vi "RydbergExpControl_2014.09.17_beta_b.vi"() -> ()   [LabVIEW 2013]
uses:
  AndorCamera/camera_controls.ctl
  <userlib>/atmcd32d.llb/AcquisitionMode_mode typedef.ctl
  <userlib>/atmcd32d.llb/TriggerMode_mode typedef.ctl
  6704/6704_static_voltages_control.ctl
  rydberg_state_machine_states.ctl
panel:
  out "Current Param Value":dbl
  out "Camera Ready":bool
  out "Exp Running":bool
  out "error out":errorcluster
  in  "Trigger Snap Mode":bool
  in  "Shutdown Experiment":bool
  in  "Start Experiment":bool
  out "Started in trigger snap":bool=TRUE
  out "Waveform Chart":dbl(graph)
  in  "Count Number?":bool
  out "Number":dbl format="%^#_6g"
  out "OD":dbl[][](graph)
  out "Atom Closeup":dbl[][](graph)
  out "Atoms - BG":dbl[][](graph)
  out "Background Image":dbl[][](graph)
  out "Atom Image":dbl[][](graph)
  in  "Tab Control":T1(tab)
  in  "Instructions":T2(array[cluster])=[{"Instruct Data"=0, "Op Code"=0, "Flags"=[TRUE, FALSE, FALSE, FALSE, FALSE, FALSE, FALSE, FALSE, FALSE, FALSE, FALSE, FALSE, FALSE, FALSE, FALSE, FALSE, FALSE, FALSE, FALSE, FALSE, FALSE, FALSE, FALSE, FALSE], "Comments"="", "Time (s)"=0.1}, {"Instruct Data"=0, "Op Code"=0, "Flags"=[FALSE, FALSE, FALSE, FALSE, FALSE, FALSE, FALSE, FALSE, FALSE, FALSE, FALSE, FALSE, FALSE, FALSE, FALSE, FALSE, FALSE, FALSE, FALSE, FALSE, FALSE, FALSE, FALSE, FALSE], "Comments"="", "Time (s)"=0.1}, {"Instruct Data"=0, "Op Code"=0, "Flags"=[TRUE, FALSE, FALSE, FALSE, FALSE, FALSE, FALSE, FALSE, FALSE, FALSE, FALSE, FALSE, FALSE, FALSE, FALSE, FALSE, FALSE, FALSE, FALSE, FALSE, FALSE, FALSE, FALSE, FALSE], "Comments"="", "Time (s)"=0.1}, {"Instruct Data"=0, "Op Code"=6, "Flags"=[FALSE, FALSE, FALSE, FALSE, FALSE, FALSE, FALSE, FALSE, FALSE, FALSE, FALSE, FALSE, FALSE, FALSE, FALSE, FALSE, FALSE, FALSE, FALSE, FALSE, FALSE, FALSE, FALSE, FALSE], "Comments"="", "Time (s)"=0.1}] {"Time (s)" format="%.3p"; "Op Code" items=["Continue", "Stop", "Loop", "End Loop", "JSR", "RTS", "Branch", "Long Delay", "Wait"]}
  in  "Parameter Nickname (no spaces)":string[](array[string])
  in  "Number of Parameters to Scan":i32=1 min=1
  in  "Channels to Change":dbl[](array[numeric])=[0.0, 0.0, 0.0]
  in  "Parameters to Change":enum16{"PulseBlaster", "Static Voltage"}[](array[ring])=[enum."Static Voltage", enum."Static Voltage", enum."Static Voltage"]
  in  "Step Sizes":dbl[](array[numeric])=[0.0, 0.0, 0.0]
  in  "Final Values":dbl[](array[numeric])=[0.0, 0.0, 0.0]
  in  "Initial Values":dbl[](array[numeric])
  in  "Scan Base Name":string
  in  "Raw_Data Folder":path
  out "Full Scan Name":string
  out "Camera Information":T3 {"VS Speed (us)" format="%.2f"}
  in  "Acquisition Parameters":T4={"Acquisition Mode"=enum."Kinetics", "Trigger Mode"=enum."External", "Frame \nTransfer"=FALSE, "Exposure Time (s)"=0.0001, "Accumulation Cycle Time (s)"=0.0, "# Accumulations"=1, "# Kinetics"=2, "Kinetic Cycle Time (s)"=0.0, "Horizontal Bin Size"=1, "Vertical Bin Size"=1} {"Vertical Bin Size" min=1; "Horizontal Bin Size" min=1; "Kinetic Cycle Time (s)" format="%.2f"; "# Kinetics" min=1; "# Accumulations" min=1; "Accumulation Cycle Time (s)" format="%.2f"; "Exposure Time (s)" format="%.2e"}
  out "Calcualted Times":T7 {"Kinetic" format="%.4f"; "Accumulate" format="%.4f"; "Exposure" format="%.4f"}
  in  "Red MOT 87 Inputs":T8={"Active Device"="6733_Red_87", "Active Channels"=[TRUE, FALSE, FALSE, FALSE, FALSE, FALSE, FALSE, FALSE], "Waveform Parameters"=[[{"Functional Form"=enum."Polynomial", "Start Voltage"=0.0, "End Voltage"=0.0, "Time"=0.0, "Degree"=1, "Sample Rate"=0.0}, {"Functional Form"=enum."Exponential", "Start Voltage"=0.0, "End Voltage"=0.0, "Time"=0.0, "Degree"=1, "Sample Rate"=0.0}, {"Functional Form"=enum."Exponential", "Start Voltage"=0.0, "End Voltage"=0.0, "Time"=0.0, "Degree"=1, "Sample Rate"=0.0}, {"Functional Form"=enum."Exponential", "Start Voltage"=0.0, "End Voltage"=0.0, "Time"=0.0, "Degree"=1, "Sample Rate"=0.0}, {"Functional Form"=enum."Exponential", "Start Voltage"=0.0, "End Voltage"=0.0, "Time"=0.0, "Degree"=1, "Sample Rate"=0.0}, {"Functional Form"=enum."Exponential", "Start Voltage"=0.0, "End Voltage"=0.0, "Time"=0.0, "Degree"=1, "Sample Rate"=0.0}], [{"Functional Form"=enum."Exponential", "Start Voltage"=0.0, "End Voltage"=0.0, "Time"=0.0, "Degree"=1, "Sample Rate"=0.0}, {"Functional Form"=enum."Exponential", "Start Voltage"=0.0, "End Voltage"=0.0, "Time"=0.0, "Degree"=1, "Sample Rate"=0.0}, {"Functional Form"=enum."Exponential", "Start Voltage"=0.0, "End Voltage"=0.0, "Time"=0.0, "Degree"=1, "Sample Rate"=0.0}, {"Functional Form"=enum."Exponential", "Start Voltage"=0.0, "End Voltage"=0.0, "Time"=0.0, "Degree"=1, "Sample Rate"=0.0}, {"Functional Form"=enum."Exponential", "Start Voltage"=0.0, "End Voltage"=0.0, "Time"=0.0, "Degree"=1, "Sample Rate"=0.0}, {"Functional Form"=enum."Exponential", "Start Voltage"=0.0, "End Voltage"=0.0, "Time"=0.0, "Degree"=1, "Sample Rate"=0.0}], [{"Functional Form"=enum."Exponential", "Start Voltage"=0.0, "End Voltage"=0.0, "Time"=0.0, "Degree"=1, "Sample Rate"=0.0}, {"Functional Form"=enum."Exponential", "Start Voltage"=0.0, "End Voltage"=0.0, "Time"=0.0, "Degree"=1, "Sample Rate"=0.0}, {"Functional Form"=enum."Exponential", "Start Voltage"=0.0, "End Voltage"=0.0, "Time"=0.0, "Degree"=1, "Sample Rate"=0.0}, {"Functional Form"=enum."Exponential", "Start Voltage"=0.0, "End Voltage"=0.0, "Time"=0.0, "Degree"=1, "Sample Rate"=0.0}, {"Functional Form"=enum."Exponential", "Start Voltage"=0.0, "End Voltage"=0.0, "Time"=0.0, "Degree"=1, "Sample Rate"=0.0}, {"Functional Form"=enum."Exponential", "Start Voltage"=0.0, "End Voltage"=0.0, "Time"=0.0, "Degree"=1, "Sample Rate"=0.0}], [{"Functional Form"=enum."Exponential", "Start Voltage"=0.0, "End Voltage"=0.0, "Time"=0.0, "Degree"=1, "Sample Rate"=0.0}, {"Functional Form"=enum."Exponential", "Start Voltage"=0.0, "End Voltage"=0.0, "Time"=0.0, "Degree"=1, "Sample Rate"=0.0}, {"Functional Form"=enum."Exponential", "Start Voltage"=0.0, "End Voltage"=0.0, "Time"=0.0, "Degree"=1, "Sample Rate"=0.0}, {"Functional Form"=enum."Exponential", "Start Voltage"=0.0, "End Voltage"=0.0, "Time"=0.0, "Degree"=1, "Sample Rate"=0.0}, {"Functional Form"=enum."Exponential", "Start Voltage"=0.0, "End Voltage"=0.0, "Time"=0.0, "Degree"=1, "Sample Rate"=0.0}, {"Functional Form"=enum."Exponential", "Start Voltage"=0.0, "End Voltage"=0.0, "Time"=0.0, "Degree"=1, "Sample Rate"=0.0}], [{"Functional Form"=enum."Exponential", "Start Voltage"=0.0, "End Voltage"=0.0, "Time"=0.0, "Degree"=1, "Sample Rate"=0.0}, {"Functional Form"=enum."Exponential", "Start Voltage"=0.0, "End Voltage"=0.0, "Time"=0.0, "Degree"=1, "Sample Rate"=0.0}, {"Functional Form"=enum."Exponential", "Start Voltage"=0.0, "End Voltage"=0.0, "Time"=0.0, "Degree"=1, "Sample Rate"=0.0}, {"Functional Form"=enum."Exponential", "Start Voltage"=0.0, "End Voltage"=0.0, "Time"=0.0, "Degree"=1, "Sample Rate"=0.0}, {"Functional Form"=enum."Exponential", "Start Voltage"=0.0, "End Voltage"=0.0, "Time"=0.0, "Degree"=1, "Sample Rate"=0.0}, {"Functional Form"=enum."Exponential", "Start Voltage"=0.0, "End Voltage"=0.0, "Time"=0.0, "Degree"=1, "Sample Rate"=0.0}], [{"Functional Form"=enum."Exponential", "Start Voltage"=0.0, "End Voltage"=0.0, "Time"=0.0, "Degree"=1, "Sample Rate"=0.0}, {"Functional Form"=enum."Exponential", "Start Voltage"=0.0, "End Voltage"=0.0, "Time"=0.0, "Degree"=1, "Sample Rate"=0.0}, {"Functional Form"=enum."Exponential", "Start Voltage"=0.0, "End Voltage"=0.0, "Time"=0.0, "Degree"=1, "Sample Rate"=0.0}, {"Functional Form"=enum."Exponential", "Start Voltage"=0.0, "End Voltage"=0.0, "Time"=0.0, "Degree"=1, "Sample Rate"=0.0}, {"Functional Form"=enum."Exponential", "Start Voltage"=0.0, "End Voltage"=0.0, "Time"=0.0, "Degree"=1, "Sample Rate"=0.0}, {"Functional Form"=enum."Exponential", "Start Voltage"=0.0, "End Voltage"=0.0, "Time"=0.0, "Degree"=1, "Sample Rate"=0.0}], [{"Functional Form"=enum."Exponential", "Start Voltage"=0.0, "End Voltage"=0.0, "Time"=0.0, "Degree"=1, "Sample Rate"=0.0}, {"Functional Form"=enum."Exponential", "Start Voltage"=0.0, "End Voltage"=0.0, "Time"=0.0, "Degree"=1, "Sample Rate"=0.0}, {"Functional Form"=enum."Exponential", "Start Voltage"=0.0, "End Voltage"=0.0, "Time"=0.0, "Degree"=1, "Sample Rate"=0.0}, {"Functional Form"=enum."Exponential", "Start Voltage"=0.0, "End Voltage"=0.0, "Time"=0.0, "Degree"=1, "Sample Rate"=0.0}, {"Functional Form"=enum."Exponential", "Start Voltage"=0.0, "End Voltage"=0.0, "Time"=0.0, "Degree"=1, "Sample Rate"=0.0}, {"Functional Form"=enum."Exponential", "Start Voltage"=0.0, "End Voltage"=0.0, "Time"=0.0, "Degree"=1, "Sample Rate"=0.0}], [{"Functional Form"=enum."Exponential", "Start Voltage"=0.0, "End Voltage"=0.0, "Time"=0.0, "Degree"=1, "Sample Rate"=0.0}, {"Functional Form"=enum."Exponential", "Start Voltage"=0.0, "End Voltage"=0.0, "Time"=0.0, "Degree"=1, "Sample Rate"=0.0}, {"Functional Form"=enum."Exponential", "Start Voltage"=0.0, "End Voltage"=0.0, "Time"=0.0, "Degree"=1, "Sample Rate"=0.0}, {"Functional Form"=enum."Exponential", "Start Voltage"=0.0, "End Voltage"=0.0, "Time"=0.0, "Degree"=1, "Sample Rate"=0.0}, {"Functional Form"=enum."Exponential", "Start Voltage"=0.0, "End Voltage"=0.0, "Time"=0.0, "Degree"=1, "Sample Rate"=0.0}, {"Functional Form"=enum."Exponential", "Start Voltage"=0.0, "End Voltage"=0.0, "Time"=0.0, "Degree"=1, "Sample Rate"=1.0}]], "Active Phases"=[TRUE, FALSE, FALSE, FALSE, FALSE, FALSE], "Phase Times"=[0.001], "Trigger Channel"="/6733_Red_87/PFI0"} {"Phase Times" format="%.0p"; "Waveform Parameters"."Degree" min=1}
  in  "6704 Static Voltage Settings":T9={"Device Name"="6704_Static", "Voltages"=[5.0, 0.0, 0.0, 0.0, 0.0, 0.0, 0.0, 0.0, 0.0, 0.0, 0.0, 0.0, 0.0, 0.0, 0.0, 0.0]}
  out "Andor Initialization Error Codes":T10
  out "Acq. Error Codes":T11
  out "Tree":string(tree)
  # "(1) 461 MOT beams"
  # "(2) Imaging AOM 1"
  # "(3) Imaging AOM 2"
  # "(4) Camera"
  # "(5) Zeeman shutter"
  # "(6) Repumper shutter"
  # "(7) 461 MOT coils"
  # "(8) 689 MOT coils"
  # "(9) 87 Sr Red MOT Trig"
  # "(10) Blue MOT Shutter"
  # "(11) Red AOM"
  # "(12) Sat Abs Current Switch"
  # "(13) Zeeman MOSFET"
  # "1"
  # "2"
  # "3"
  # "4"
  # "5"
  # "6"
  # "7"
  # "8"
  # "9"
  # "10"
  # "11"
  # "12"
  # "13"
  # "14"
  # "15"
  # "16"
  # "17"
  # "18"
  # "19"
  # "20"
  # "21"
  # "22"
  # "23"
  # "24"
  # "Conversion formulae to be added"
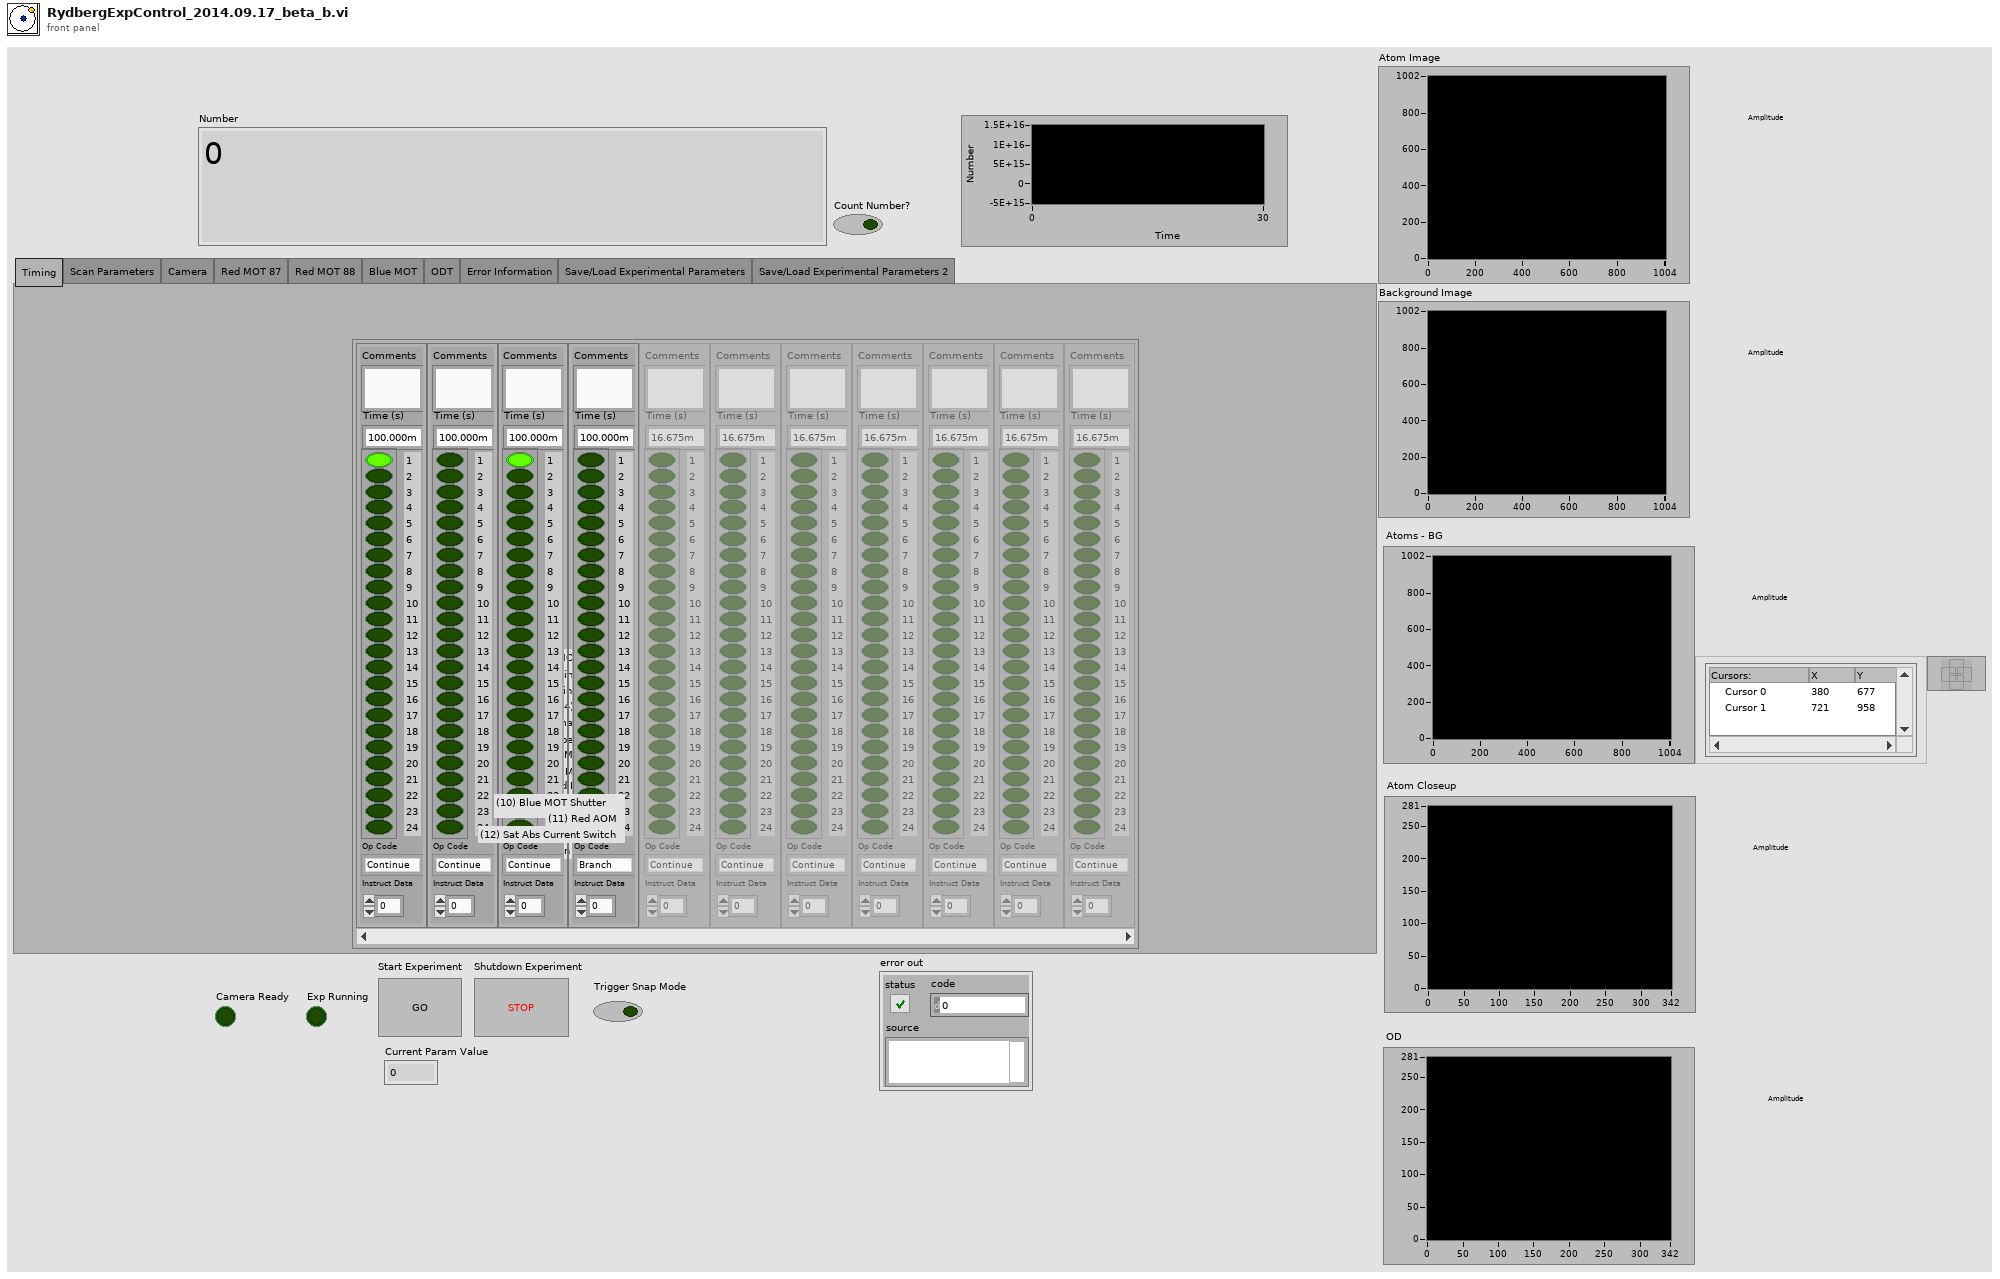
[diagram p1: front panel]
types:
  T1 = enum32{"Timing", "Scan Parameters", "Camera", "Red MOT 87", "Red MOT 88", "Blue MOT", "ODT", "Error Information", "Save/Load Experimental Parameters", "Save/Load Experimental Parameters 2"}
  T2 = cluster{"Instruct Data":i32, "Op Code":i32, "Flags":bool[], "Comments":string, "Time (s)":dbl}[]
  T3 = cluster{"xpixels":i32, "ypixels":i32, "# VS Speeds":i32, "VS Speed (us)":sgl, "Temperature Stable":bool, "Temperature (C)":i32}
  T4 = typedef "camera_controls.ctl" = cluster{"Acquisition Mode":T5, "Trigger Mode":T6, "Frame \nTransfer":bool, "Exposure Time (s)":sgl, "Accumulation Cycle Time (s)":sgl, "# Accumulations":i32, "# Kinetics":i32, "Kinetic Cycle Time (s)":sgl, "Horizontal Bin Size":i32, "Vertical Bin Size":i32}
  T5 = typedef "AcquisitionMode_mode typedef.ctl" = enum16{"Reserved (0)", "Single Scan", "Accumulate", "Kinetics", "Fast Kinetics", "Run Till Abort", "Reserved (6)", "Reserved (7)", "Reserved (8)", "Time Delayed Integration"}
  T6 = typedef "TriggerMode_mode typedef.ctl" = enum16{"Internal", "External", "N/A (2)", "N/A (3)", "N/A (4)", "N/A (5)", "External Start", "External Exposure (Bulb)", "N/A (8)", "External FVB EM", "Software", "N/A (11)", "External Charge Shifting"}
  T7 = cluster{"Exposure":sgl, "Accumulate":sgl, "Kinetic":sgl}
  T8 = cluster{"Active Device":string, "Active Channels":bool[], "Waveform Parameters":cluster{"Functional Form":enum16{"Polynomial", "Exponential"}, "Start Voltage":dbl, "End Voltage":dbl, "Time":dbl, "Degree":i8, "Sample Rate":dbl}[][], "Active Phases":bool[], "Phase Times":dbl[], "Trigger Channel":tag}
  T9 = typedef "6704_static_voltages_control.ctl" = cluster{"Device Name":string, "Voltages":dbl[]}
  T10 = cluster{"Initalize Error Code":u32, "GetDetector Error Code":u32, "Get#VSSpeeds Error Code":u32, "Set VS Speed Error":u32, "CoolerOn Error Code":u32, "GetTemperature Error Code":u32, "Shutdown Error Code":u32}
  T11 = cluster{"Set Acq. Mode Error":u32, "Set Trigger Mode Error":u32, "Set FT Error Code":u32, "Set Exposure Time Error Code":u32, "Set Accum Time Error":u32, "Set # Accum Error":u32, "Set # Kinetics Error":u32, "SetKinCycleTime Error":u32}
  T12 = typedef "rydberg_state_machine_states.ctl" = enum16{"Initialize", "Idle", "Experiment Running", "Trigger Snap Mode", "Scan Mode", "Load Experiment", "Shutdown"}
  T13 = cluster{"6704 Static Voltage Settings":T9, "Instructions":cluster{"Instruct Data":i32, "Op Code":i32, "Flags":bool[], "Comments":string, "Time (s)":dbl}[], "Red MOT 87 Inputs":cluster{"Active Device":string, "Active Channels":bool[], "Waveform Parameters":cluster{"Functional Form":enum16{"Polynomial", "Exponential"}, "Start Voltage":dbl, "End Voltage":dbl, "Time":dbl, "Degree":i8, "Sample Rate":dbl}[][], "Active Phases":bool[], "Phase Times":dbl[], "Trigger Channel":tag}}
  T14 = cluster{"Initial Values":refnum<vi>, "Channels to Change":refnum<vi>, "Final Values":refnum<vi>, "Step Sizes":refnum<vi>}
  T15 = typedef "LVCursorListTypeDef.ctl" = cluster{"Name":string, "Color":u32, "Style":u8, "Point Style":u8, "Name Visible":bool, "Allow Drag":bool, "Cursor Mode":u32, "Plot":i32, "Index":i32, "Position":cluster{"X":dbl, "Y":dbl}, "X Scale":u32, "Y Scale":u32, "Watch Plots":i32[], "Watch All Plots":bool, "Plot Area":i32, "Label Offset":cluster{"X":dbl, "Y":dbl}}[]
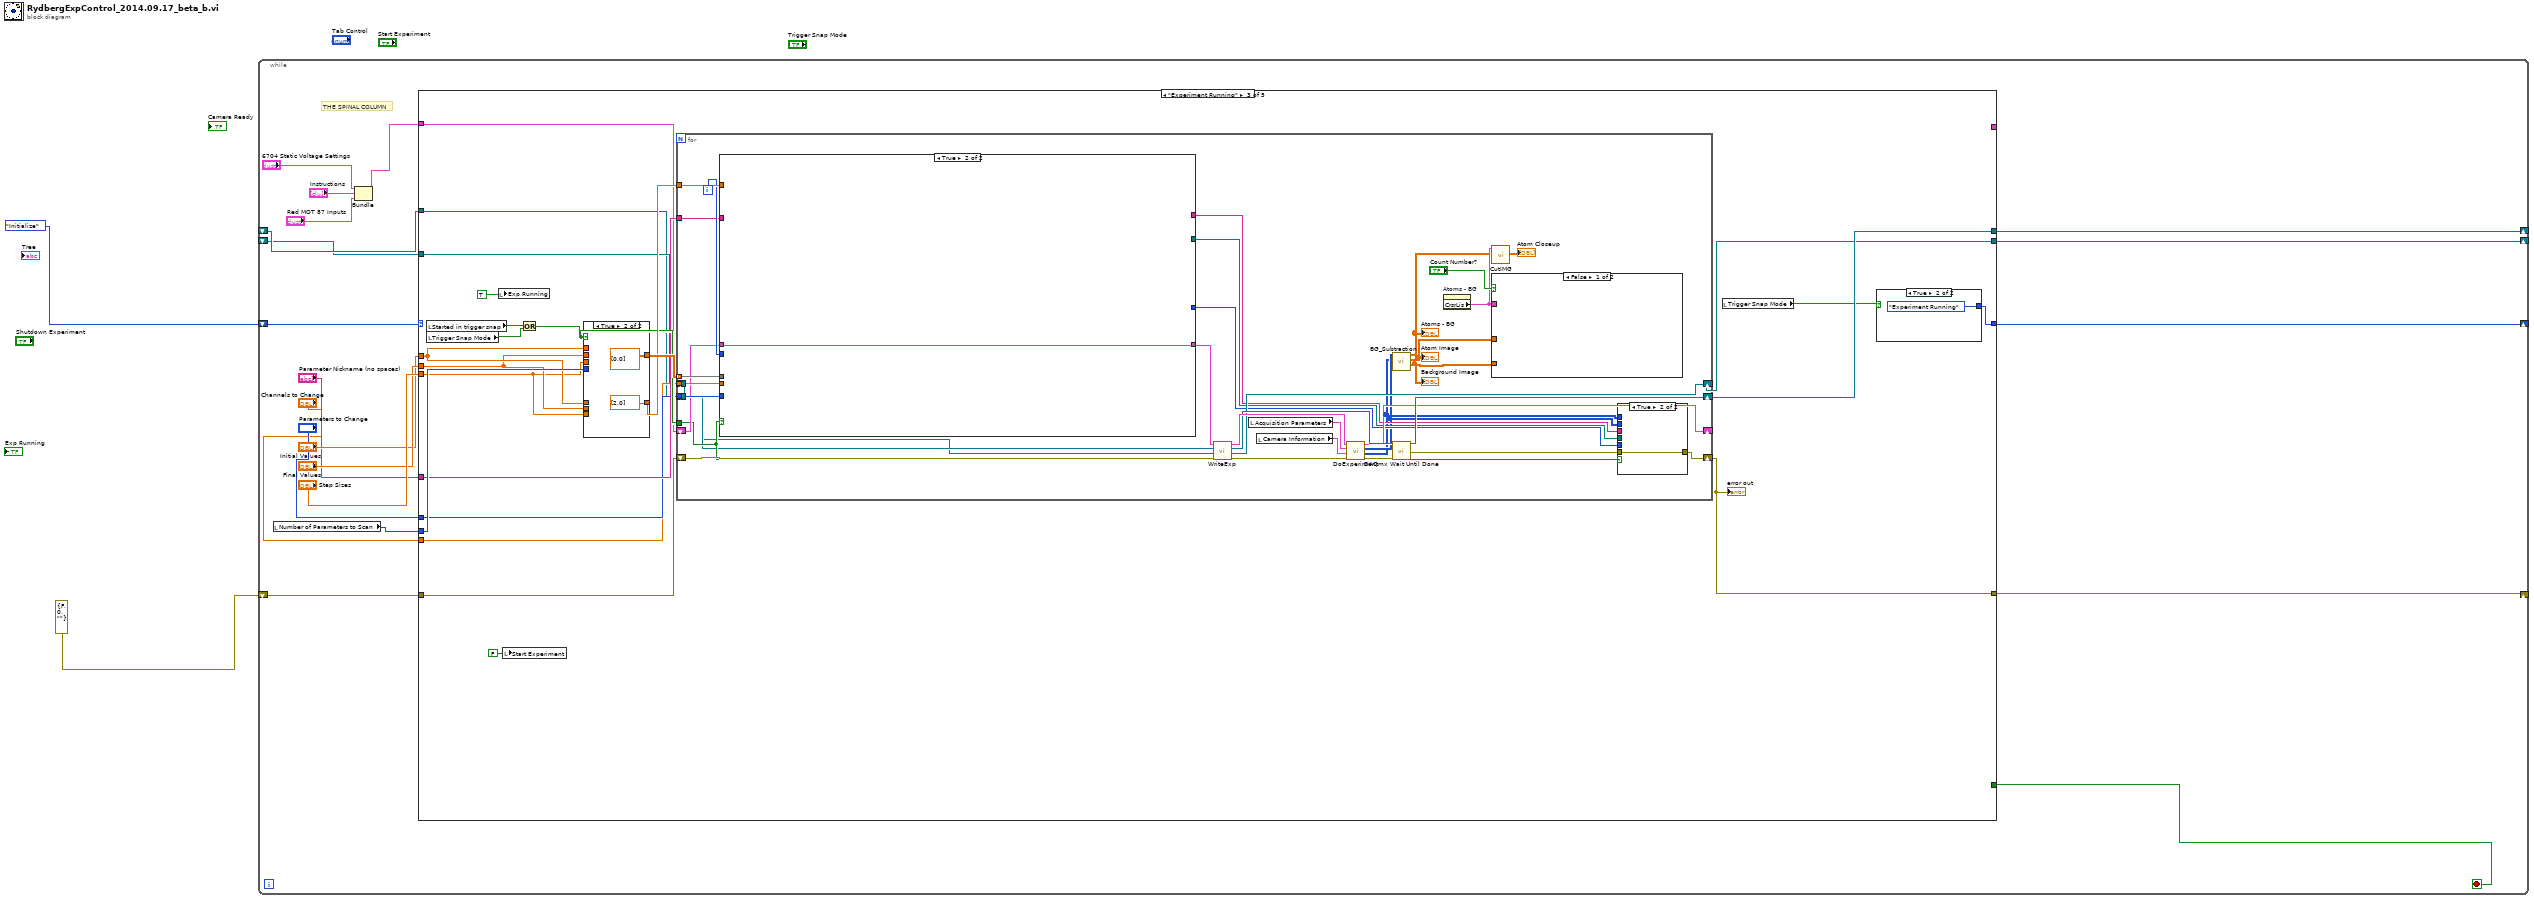
[diagram p0: block diagram]
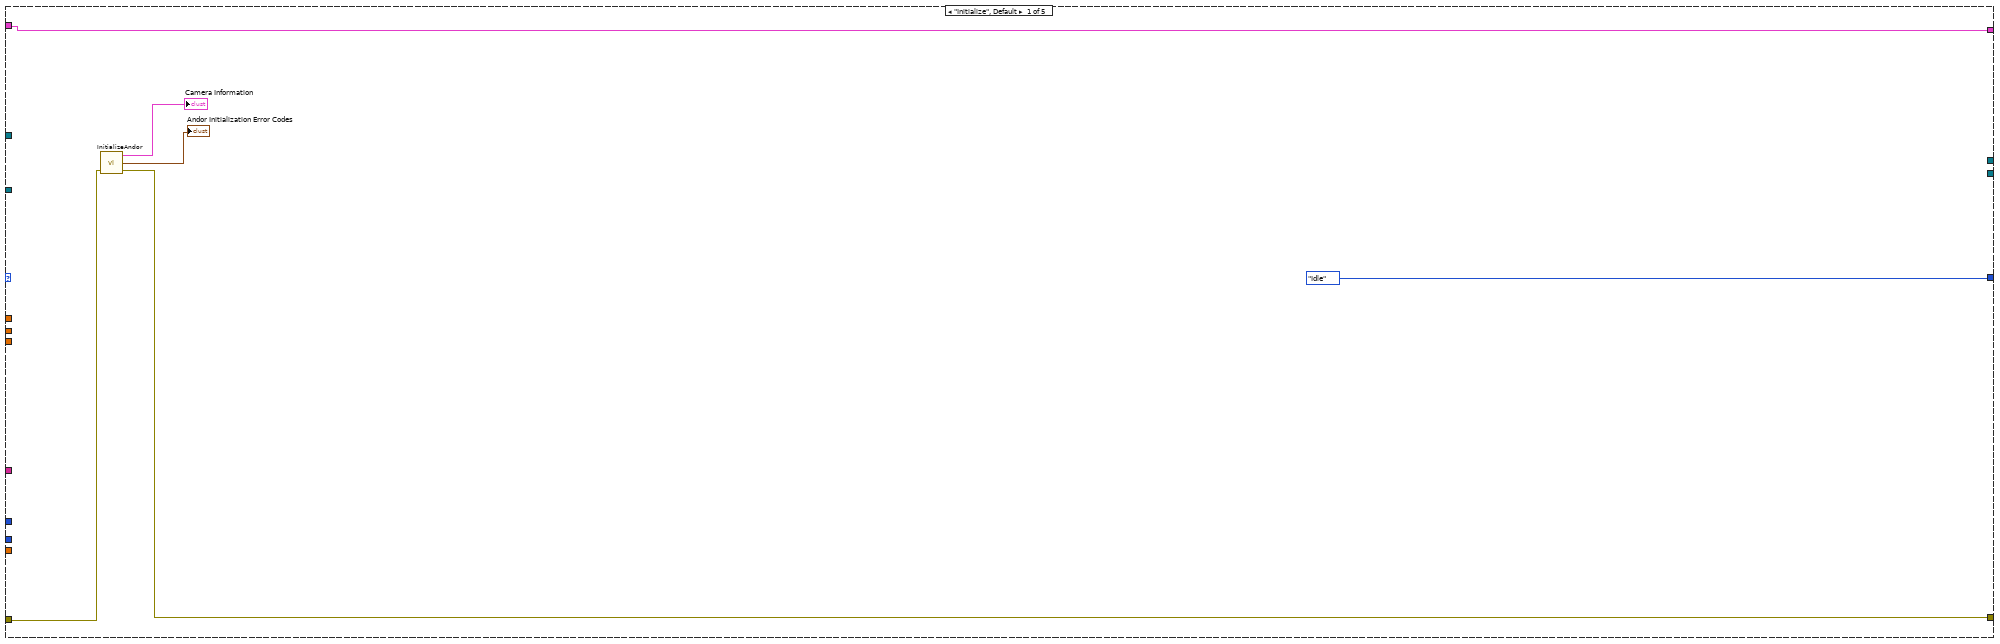
[diagram p2: hidden frame]
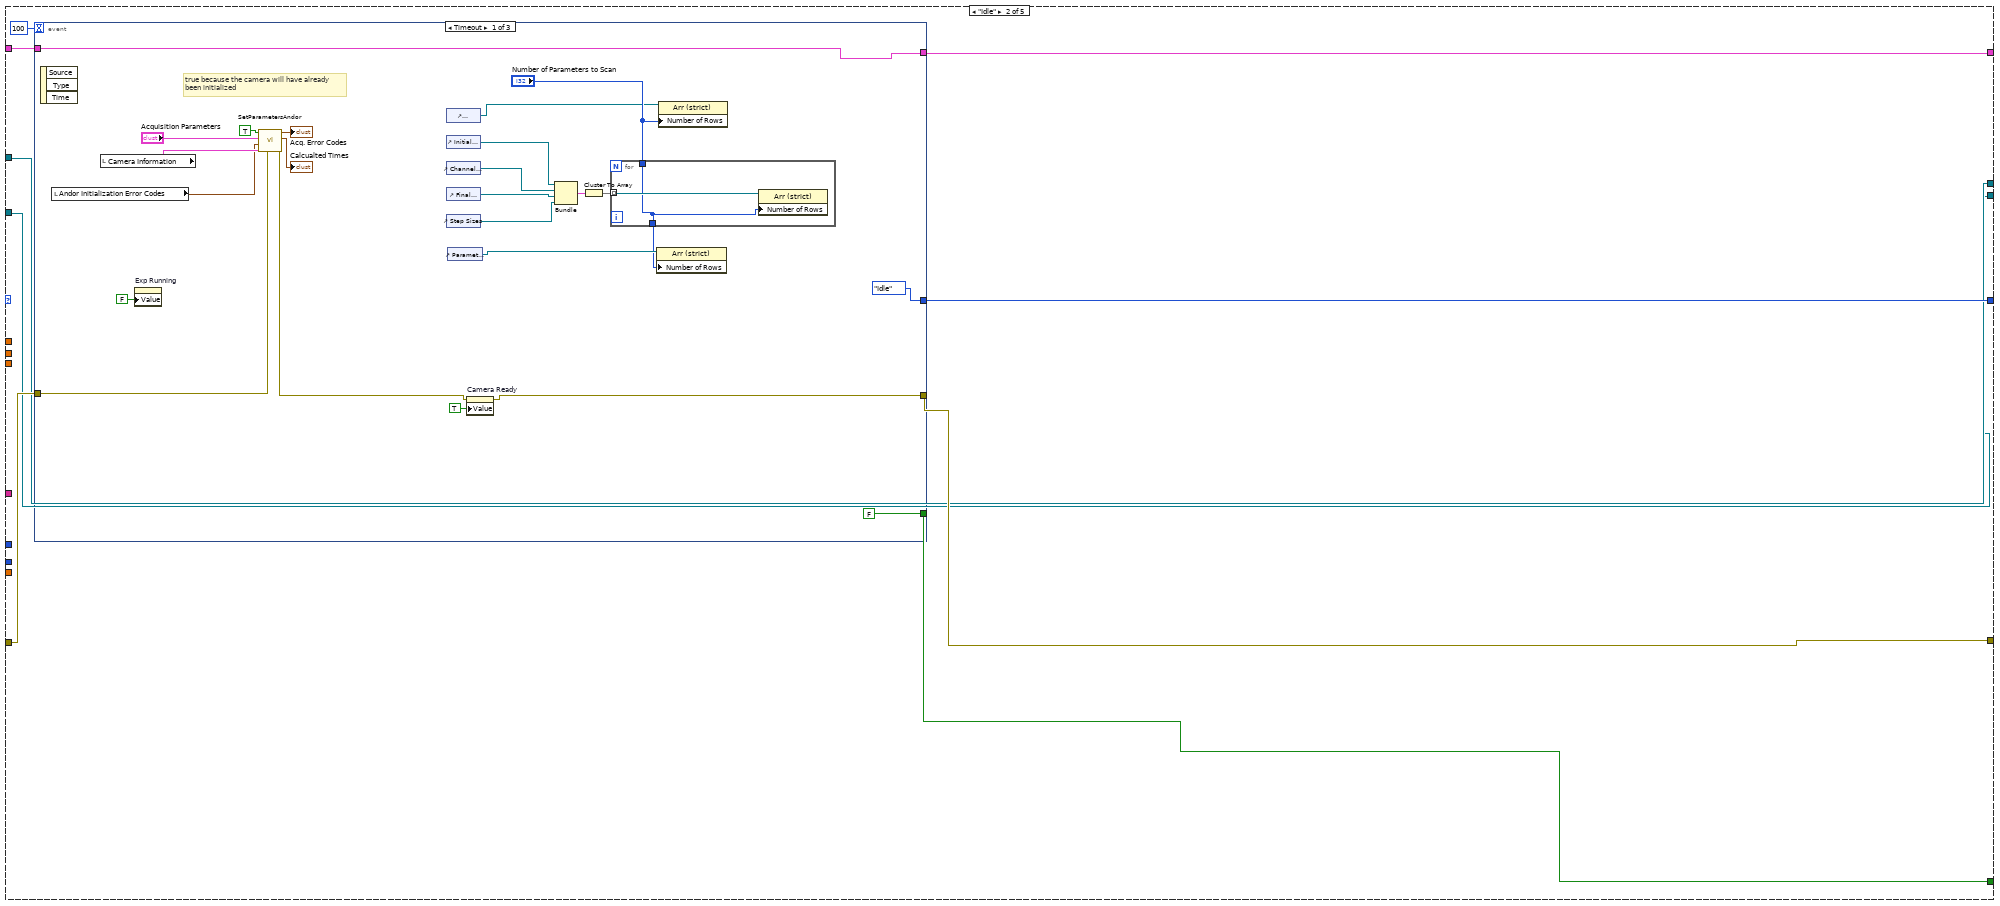
[diagram p3: hidden frame]
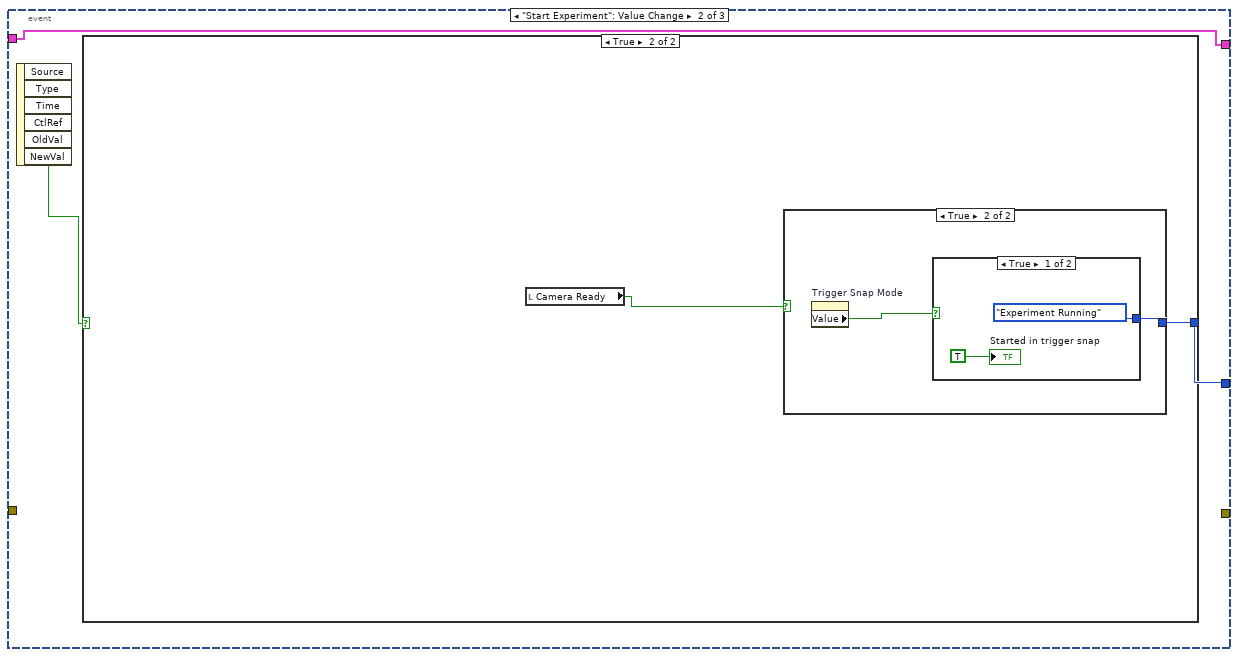
[diagram p4: hidden frame]
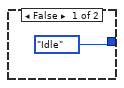
[diagram p5: hidden frame]
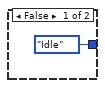
[diagram p6: hidden frame]
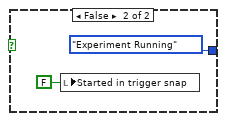
[diagram p7: hidden frame]
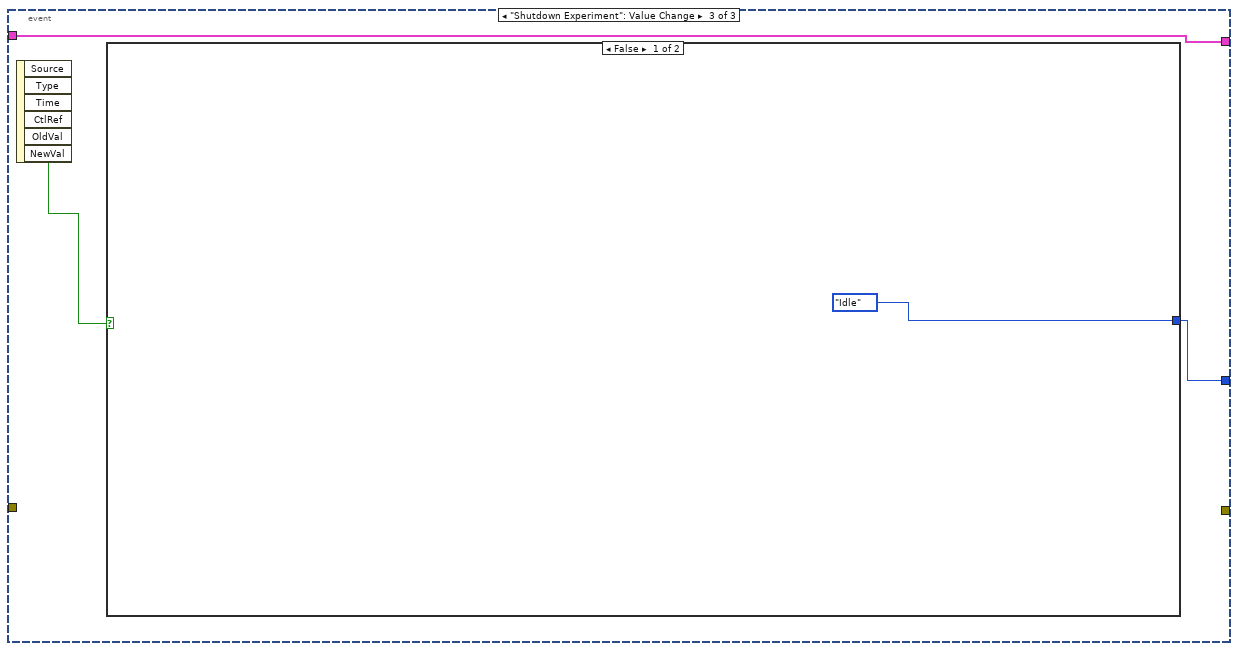
[diagram p8: hidden frame]
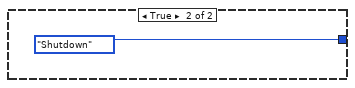
[diagram p9: hidden frame]
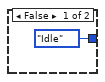
[diagram p10: hidden frame]
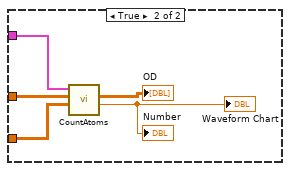
[diagram p11: hidden frame]
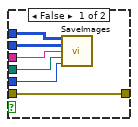
[diagram p12: hidden frame]
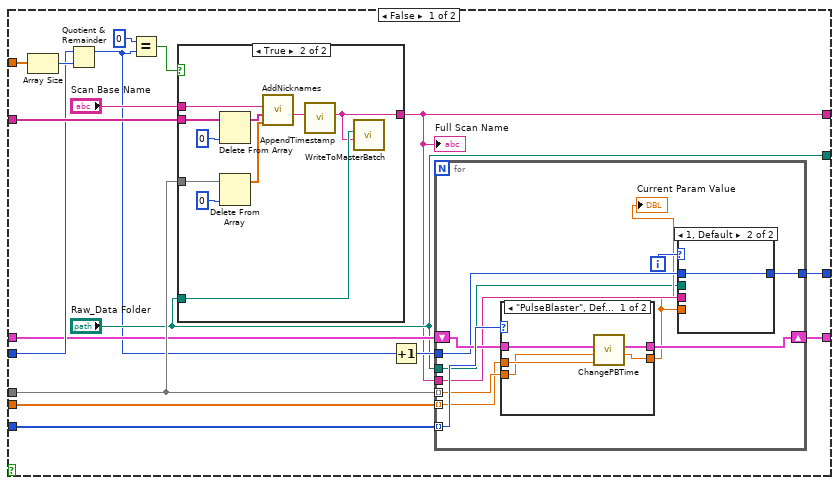
[diagram p13: hidden frame]
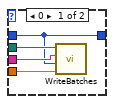
[diagram p14: hidden frame]
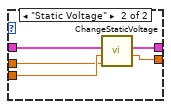
[diagram p15: hidden frame]
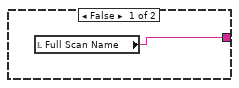
[diagram p16: hidden frame]
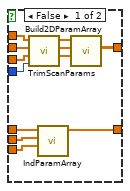
[diagram p17: hidden frame]
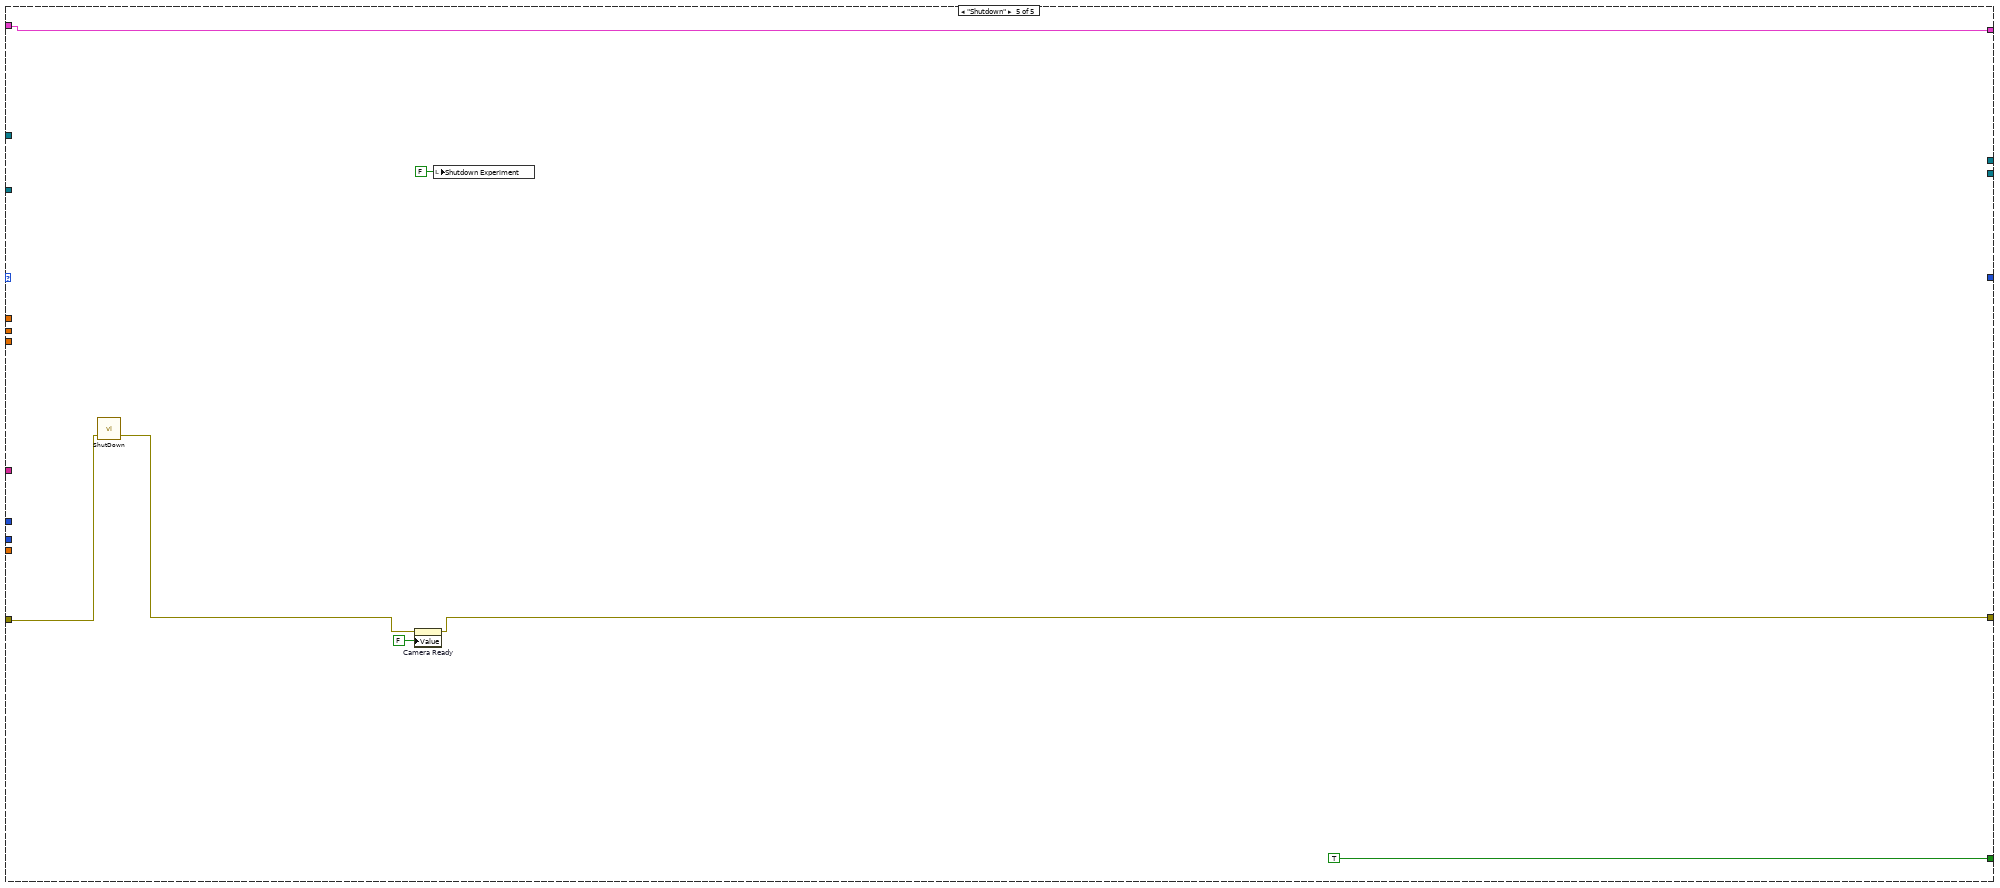
[diagram p19: hidden frame]
diagram:
  n1 = while {
    shift-right: [w19] -> _
    shift-left: rydberg_state_machine_states."Initialize" -> [w22]
    shift-right: [w20] -> _
    shift-left: errorcluster {"status"=FALSE, "code"=0, "source"=""} ("error constant") -> [w21]
    shift-right: [w13] -> _
    shift-left: _ -> [w12]
    shift-right: [w11] -> _
    shift-left: _ -> [w10]
    stop <- w18 stop-if-true
    # "THE SPINAL COLUMN"
    n2 = local read "Number of Parameters to Scan"() -> (w9:i32)
    n3 = Bundle("6704 Static Voltage Settings"="6704 Static Voltage Settings", "Instructions"="Instructions", "Red MOT 87 Inputs"="Red MOT 87 Inputs") -> (w14:T13)  [unwired: 1 in]
    n4 = case shown="\"Experiment Running\"" w22 {
      tunnel: w21 -> [w28 w37 w91 _ w229]
      tunnel: [w25 w33 w88 _ w224] -> w20
      tunnel: [rydberg_state_machine_states."Idle" w35 w84 _ _] -> w19
      tunnel: [_ w34 _ _ TRUE] -> w18
      tunnel: [w23 w32 _ w222 w226] -> _
      tunnel: w14 -> [w23 w31 w92 w222 w226]
      tunnel: [_ w30 w90 _ _] -> w13
      tunnel: w12 -> [_ w30 w86 _ _]
      tunnel: [_ w29 w89 _ _] -> w11
      tunnel: w10 -> [_ w29 w87 _ _]
      tunnel: w9 -> [_ _ w102 _ _]
      tunnel: "Step Sizes" -> [_ _ w98 _ _]
      tunnel: "Final Values" -> [_ _ w99 _ _]
      tunnel: "Initial Values" -> [_ _ w100 _ _]
      tunnel: "Parameter Nickname (no spaces)" -> [_ _ w95 _ _]
      tunnel: "Parameters to Change" -> [_ _ w94 _ _]
      tunnel: "Channels to Change" -> [_ _ w93 _ _]
      frame "Initialize", Default {
        n5 = call "InitializeAndor.vi"("Error In"=w28) -> ("error out"=w25:errorcluster, "Andor Initialization Error Codes"=→"Andor Initialization Error Codes":T10, "Camera Information"=→"Camera Information":T3)  [unwired: 2 in]
      }
      frame "Idle" {
        n6 = event shown="[0] Timeout" {
          selector: _ -> [_ _ _]
          dyn-events: _ -> [_ _ _]
          timeout: 100 -> [_ _ _]
          tunnel: w37 -> [w55 _ _]
          tunnel: [rydberg_state_machine_states."Idle" w65 w78] -> w35
          tunnel: [FALSE _ _] -> w34
          tunnel: [w49 _ _] -> w33
          tunnel: [w52 w64 w77] -> w32
          tunnel: w31 -> [w52 w64 w77]
          event Timeout {
            # "true because the camera will have already\nbeen initialized"
            n7 = event-data() -> ()  [unwired: 1 in, 3 out]
            n8 = local read "Andor Initialization Error Codes"() -> (w54:T10)
            n9 = local read "Camera Information"() -> (w57:T3)
            n10 = property on="Exp Running" class="Bool (strict)"("Value"=FALSE ("Exp Running")) -> ()  [unwired: 2 in, 2 out]
            n11 = call "SetParametersAndor.vi"("Error In"=w55, "Camera Information"=w57, "Andor Initialization Error Codes"=w54, "Acquisition Parameters"="Acquisition Parameters", "Pre Initialized?"=TRUE) -> ("error out"=w50:errorcluster, "Calcualted Times"=→"Calcualted Times":T7, "Acq. Error Codes"=→"Acq. Error Codes":T11)  [unwired: 4 in]
            n12 = control-ref of="Parameters to Change"() -> (w40:refnum<vi>)
            n13 = control-ref of="Initial Values"() -> (w47:refnum<vi>)
            n14 = control-ref of="Channels to Change"() -> (w46:refnum<vi>)
            n15 = control-ref of="Final Values"() -> (w45:refnum<vi>)
            n16 = control-ref of="Step Sizes"() -> (w44:refnum<vi>)
            n17 = control-ref of="Parameter Nickname (no spaces)"() -> (w39:refnum<vi>)
            n18 = property on="Camera Ready" class="Bool (strict)"(error in=w50, "Value"=TRUE ("Camera Ready")) -> (error out=w49:errorcluster)  [unwired: 1 in, 1 out]
            n19 = Bundle("Initial Values"=w47, "Channels to Change"=w46, "Final Values"=w45, "Step Sizes"=w44) -> (w43:T14)  [unwired: 1 in]
            n20 = Cluster To Array(cluster=w43) -> (array=w42:refnum<vi>[])
            n21 = for {
              tunnel: w42 -> [w63] mode=indexing
              tunnel: "Number of Parameters to Scan" -> [w62]
              tunnel: [w62] -> w38
              n22 = property class="Arr (strict)"(reference=w63, "Number of Rows"=w62) -> ()  [unwired: 1 in, 2 out]
            }
            n23 = property class="Arr (strict)"(reference=w39, "Number of Rows"=w38) -> ()  [unwired: 1 in, 2 out]
            n24 = property class="Arr (strict)"(reference=w40, "Number of Rows"="Number of Parameters to Scan") -> ()  [unwired: 1 in, 2 out]
          }
          event "Start Experiment": Value Change {
            n25 = event-data() -> ("NewVal"=w66:bool)  [unwired: 1 in, 5 out]
            n26 = case shown="True" w66 {
              tunnel: [rydberg_state_machine_states."Idle" w69] -> w65
              frame False {
              }
              frame True {
                n27 = local read "Camera Ready"() -> (w68:bool)
                n28 = case shown="True" w68 {
                  tunnel: [rydberg_state_machine_states."Idle" w72] -> w69
                  frame False {
                  }
                  frame True {
                    n29 = property on="Trigger Snap Mode" class="Bool (strict)"() -> ("Value"=w71:bool)  [unwired: 2 in, 2 out]
                    n30 = case shown="True" w71 {
                      tunnel: [rydberg_state_machine_states."Experiment Running" rydberg_state_machine_states."Experiment Running"] -> w72
                      frame True {
                        "Started in trigger snap" <- TRUE
                      }
                      frame False {
                        n31 = local write "Started in trigger snap"(FALSE ("Started in trigger snap")) -> ()
                      }
                    }
                  }
                }
              }
            }
          }
          event "Shutdown Experiment": Value Change {
            n32 = event-data() -> ("NewVal"=w79:bool)  [unwired: 1 in, 5 out]
            n33 = case shown="False" w79 {
              tunnel: [rydberg_state_machine_states."Idle" rydberg_state_machine_states."Shutdown"] -> w78
              frame False {
              }
              frame True {
              }
            }
          }
        }
      }
      frame "Experiment Running" {
        n34 = local read "Started in trigger snap"() -> (w103:bool)
        n35 = local read "Trigger Snap Mode"() -> (w104:bool)
        n36 = local write "Exp Running"(TRUE) -> ()
        n37 = local write "Start Experiment"(FALSE ("Start Experiment")) -> ()
        n38 = Or(x=w103, y=w104) -> (x .or. y?=w96:bool)
        n39 = case shown="True" w96 {
          tunnel: w102 -> [w219 _]
          tunnel: w98 -> [w218 _]
          tunnel: w99 -> [w217 _]
          tunnel: w100 -> [w216 _]
          tunnel: [w212 dbl[][] [[0.0]] ("Parameter Array")] -> w101
          tunnel: w100 -> [w211 _]
          tunnel: w99 -> [w210 _]
          tunnel: w98 -> [w209 _]
          tunnel: [w208 dbl[] [2.0] ("Array")] -> w97
          frame False {
            n40 = call "TrimScanParams.vi"("Parameters to change"=w219, "Step Sizes"=w218, "Final Values"=w217, "Initial Values"=w216) -> ("Step Sizes Out"=w213:dbl[], "Final Values Out"=w214:dbl[], "Initial Values Out"=w215:dbl[])  [unwired: 5 in]
            n41 = call "IndParamArray.vi"("Step Sizes"=w209, "Final Values"=w210, "Initial Values"=w211) -> ("Array"=w208:dbl[])  [unwired: 8 in]
            n42 = call "Build2DParamArray.vi"("Step Sizes"=w213, "Final Values"=w214, "Initial Values"=w215) -> ("Parameter Array"=w212:dbl[][])  [unwired: 8 in]
          }
          frame True {
          }
        }
        n43 = for {
          tunnel: w101 -> [w137] mode=indexing
          tunnel: w97 -> [w140]
          tunnel: w96 -> [w120]
          tunnel: w95 -> [w138]
          tunnel: w94 -> [w136]
          tunnel: w93 -> [w135]
          shift-right: [w124] -> _
          shift-left: w92 -> [w134]
          shift-right: [w122] -> w88
          shift-left: w91 -> [w133]
          shift-right: [w129] -> w89
          shift-left: w87 -> [w108]
          shift-right: [w128] -> w90
          shift-left: w86 -> [w107]
          i -> [w139]
          n44 = case shown="True" w120 {
            tunnel: w140 -> [w169 _]
            tunnel: w139 -> [w162 _]
            tunnel: w138 -> [w166 _]
            tunnel: w137 -> [w161 _]
            tunnel: w136 -> [w164 _]
            tunnel: w135 -> [w163 _]
            tunnel: w134 -> [w159 w207]
            tunnel: [w158 w207] -> w127
            tunnel: [w156 _] -> w117
            tunnel: ["Raw_Data Folder" _] -> w119
            tunnel: [w154 _] -> w118
            frame False {
              n45 = Array Size(array=w169) -> (size(s)=w168:i32)
              n46 = Quotient & Remainder(x=w162, y=w168) -> (x-y*floor(x/y)=w153:i32)  [unwired: 1 out]
              n47 = Equal?(x=0, y=w153) -> (x = y?=w165:bool)
              n48 = case shown="True" w165 {
                tunnel: w166 -> [_ w199]
                tunnel: w161 -> [_ w206]
                tunnel: "Raw_Data Folder" -> [_ w202]
                tunnel: [w196 w201] -> w154
                tunnel: "Scan Base Name" -> [_ w200]
                frame False {
                  n49 = local read "Full Scan Name"() -> (w196:string)
                }
                frame True {
                  n50 = Delete From Array(array=w199, index=0) -> (array with subset deleted=w197:string[])  [unwired: 1 in, 1 out]
                  n51 = Delete From Array(array=w206, index=0) -> (array with subset deleted=w204:dbl[])  [unwired: 1 in, 1 out]
                  n52 = call "AddNicknames.vi"("Values"=w204, "Nicknames"=w197, "Base Name"=w200) -> ("Name Out"=w203:string)  [unwired: 8 in]
                  n53 = call "AppendTimestamp.vi"("String"=w203) -> ("String 2"=w201:string)  [unwired: 10 in]
                  n54 = call "WriteToMasterBatch.vi"("Scan name"=w201, "Raw_Data Folder"=w202) -> ()  [unwired: 10 in]
                }
              }
              "Full Scan Name" <- w154
              n55 = Increment(x=w153) -> (x+1=w157:i32)
              n56 = for {
                tunnel: w164 -> [w180] mode=indexing
                tunnel: w163 -> [w177] mode=indexing
                tunnel: w161 -> [w178] mode=indexing
                tunnel: w154 -> [w174]
                tunnel: w157 -> [w173]
                tunnel: "Raw_Data Folder" -> [w171]
                tunnel: [w170] -> w156
                shift-right: [w176] -> w158
                shift-left: w159 -> [w179]
                i -> [w175]
                n57 = case shown="\"PulseBlaster\", Default" w180 {
                  tunnel: w179 -> [w190 w195]
                  tunnel: w178 -> [w187 w194]
                  tunnel: w177 -> [w188 w193]
                  tunnel: [w186 w192] -> w172
                  tunnel: [w189 w191] -> w176
                  frame "PulseBlaster", Default {
                    n58 = call "ChangePBTime.vi"("Instruction to change"=w188, "Time"=w187, "Input parameters"=w190) -> ("Time out"=w186:dbl, "output parameters"=w189:T13)  [unwired: 7 in]
                  }
                  frame "Static Voltage" {
                    n59 = call "ChangeStaticVoltage.vi"("Channel to change"=w193, "Voltage"=w194, "Parameters input"=w195) -> ("Voltage out"=w192:dbl, "Parameters Output"=w191:T13)  [unwired: 7 in]
                  }
                }
                "Current Param Value" <- w172
                n60 = case shown="1, Default" w175 {
                  tunnel: w174 -> [w184 _]
                  tunnel: w173 -> [w181 w185]
                  tunnel: w172 -> [w183 _]
                  tunnel: w171 -> [w182 _]
                  tunnel: [w181 w185] -> w170
                  frame 0 {
                    n61 = call "WriteBatches.vi"("Variable Parameter Value"=w183, "Image Number"=w181, "Scan Name"=w184, "Raw Data Folder"=w182) -> ()  [unwired: 8 in]
                  }
                  frame 1, Default {
                  }
                }
              }
            }
            frame True {
            }
          }
          n62 = call "WriteExp.vi"("error in (no error)"=w133, "Control Task In"=w107, "Waveform Task In"=w108, "Experimental Control Cluster In"=w127) -> ("error out"=w131:errorcluster, "waveform task out"=w129:refnum<k21>, "counter task out"=w130:refnum<k21>, "Experimental Control Cluster Out"=w132:T13)  [unwired: 4 in]
          n63 = local read "Acquisition Parameters"() -> (w125:T4)
          n64 = local read "Camera Information"() -> (w126:T3)
          n65 = call "DoExperiment.vi"("Error In"=w131, "Camera Information 2"=w126, "Acquisition Parameters"=w125, "output cluster"=w132) -> ("error out"=w123:errorcluster, "Background Image"=w115:i32[][], "Atom Image"=w116:i32[][], "output cluster 2"=w124:T13)  [unwired: 4 in]
          n66 = call "BG_Subtraction.vi"("Background Image"=w115, "Atom Image"=w116) -> ("Background Image Out"=w109:dbl[][], "Atom Image Out"=w110:dbl[][], "Atoms - BG"=w111:dbl[][])  [unwired: 7 in]
          "Atom Image" <- w110
          "Background Image" <- w109
          "Atoms - BG" <- w111
          n67 = call <vilib>:"DAQmx Wait Until Done.vi"("task/channels in"=w130, "error in"=w123) -> ("task out"=w128:refnum<k21>, "error out"=w121:errorcluster)  [unwired: 12 in]
          n68 = property on="Atoms - BG" class="IntGraph (strict)"() -> ("CrsrLis"=w113:T15)  [unwired: 2 in, 2 out]
          n69 = call "CutIMG.vi"("Full Image In"=w111, "Cursor List"=w113) -> ("Cut Image Out"=→"Atom Closeup":dbl[][])  [unwired: 9 in]
          n70 = case shown="False" "Count Number?" {
            tunnel: w113 -> [_ w145]
            tunnel: w110 -> [_ w144]
            tunnel: w109 -> [_ w143]
            frame False {
            }
            frame True {
              n71 = call "CountAtoms.vi"("Background Image"=w143, "Atom Image"=w144, "Cursor List"=w145) -> ("Number"=→"Waveform Chart" →"Number":dbl, "OD"=→"OD":dbl[][])  [unwired: 7 in]
            }
          }
          n72 = case shown="True" w120 {
            tunnel: [w151 w152] -> w122
            tunnel: w121 -> [w151 w152]
            tunnel: w116 -> [w150 _]
            tunnel: w115 -> [w149 _]
            tunnel: w119 -> [w148 _]
            tunnel: w118 -> [w147 _]
            tunnel: w117 -> [w146 _]
            frame False {
              n73 = call "SaveImages.vi"("Background Image"=w149, "Atoms Image"=w150, "Base Filename"=w147, "Raw Data Path"=w148, "ImageNumber"=w146) -> ()  [unwired: 9 in, 2 out]
            }
            frame True {
            }
          }
        }
        "error out" <- w88
        n74 = local read "Trigger Snap Mode"() -> (w85:bool)
        n75 = case shown="True" w85 {
          tunnel: [rydberg_state_machine_states."Idle" rydberg_state_machine_states."Experiment Running"] -> w84
          frame False {
          }
          frame True {
          }
        }
      }
      frame "Load Experiment" {
      }
      frame "Shutdown" {
        n76 = call <userlib>:"ShutDown.vi"("error in (no error)"=w229) -> ("error out"=w225:errorcluster)  [unwired: 1 in, 1 out]
        n77 = property on="Camera Ready" class="Bool (strict)"(error in=w225, "Value"=FALSE ("Camera Ready")) -> (error out=w224:errorcluster)  [unwired: 1 in, 1 out]
        n78 = local write "Shutdown Experiment"(FALSE ("Shutdown Experiment")) -> ()
      }
    }
  }
